vi "asynchronous safe state.vi"(9 "Module Info In":T1, 11 "Engine Tags In":T5) -> (1 "Module Info Out":T1, 3 "Engine Tags Out":T5)   [LabVIEW 2013, in "Standard Engine Runtime.lvclass"]
uses:
  Standard Engine Runtime.lvclass
  <vilib>/NI/Tag Bus/table/data table.ctl
  async execution info.ctl
  asynchronous process data.ctl
  async command notification.ctl
  <vilib>/NI/Tag Bus Module Framework/runtime/execution settings.ctl
  async error info.ctl
  <vilib>/NI/Tag Bus Module Framework/runtime/error classification.ctl
  Data Table with Transfer Spec.ctl
  <vilib>/NI/Tag Bus/table/transfer specification.ctl
  <vilib>/NI/Tag Bus/tag/Data Type.ctl
  Configuration/Module Decimation.ctl
  Configuration/Module Error Configuration.ctl
  Configuration/Error Actions By Category.ctl
  Configuration/Error Actions.ctl
  <vilib>/NI/Tag Bus/table/data table.lvlib
  <vilib>/NI/Tag Bus/tag/tag descriptor.lvclass
  Configuration/Standard Engine Configuration.lvclass
  <vilib>/NI/Tag Bus Module Framework/runtime/TBM module execution interface.lvclass
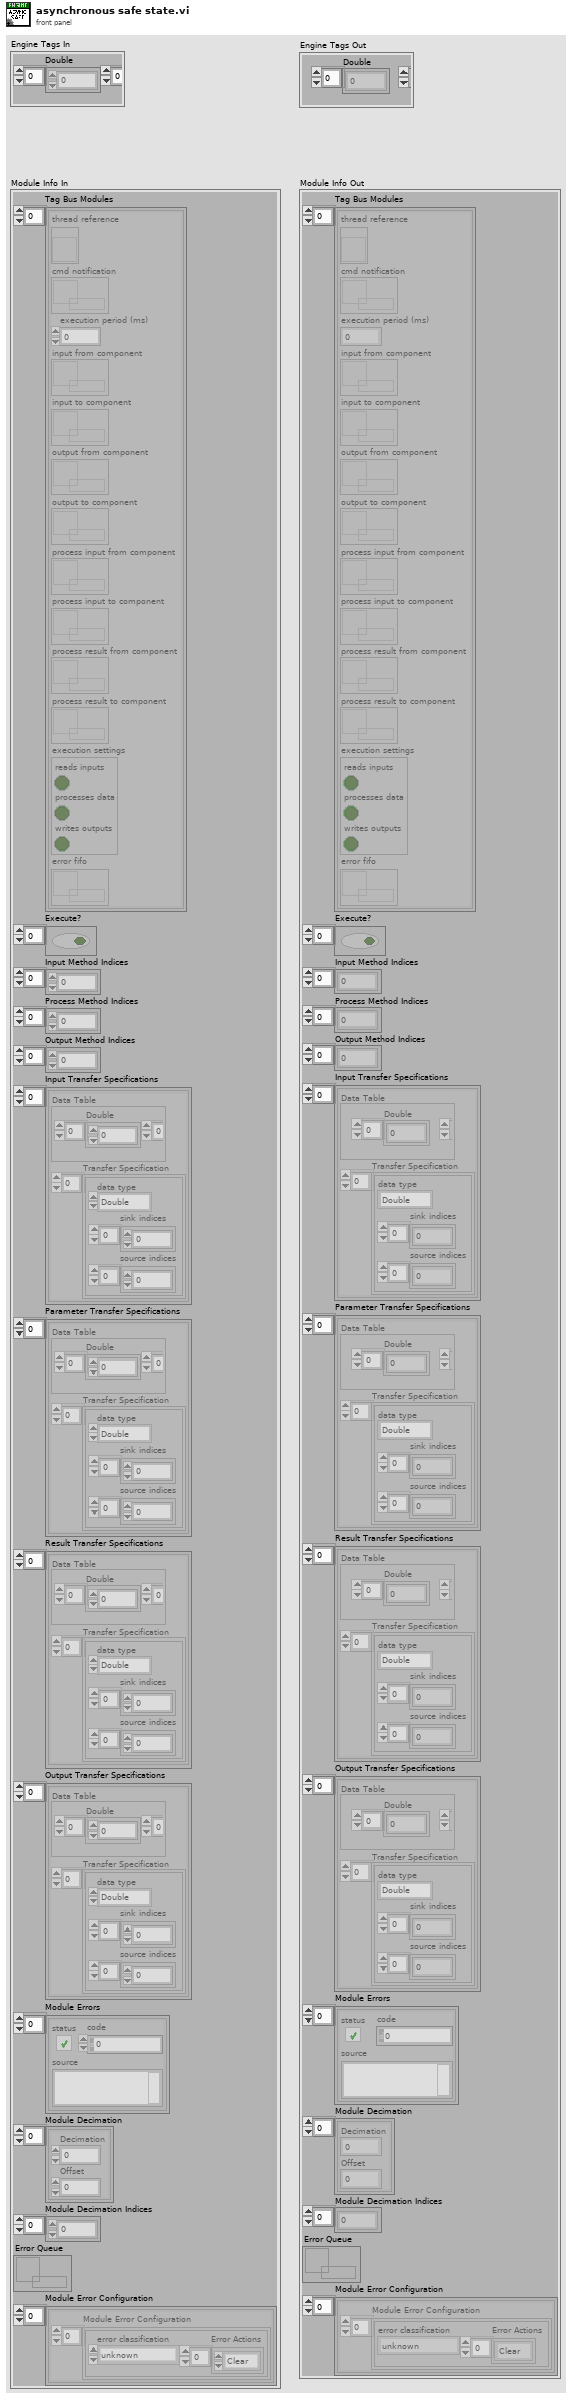
[diagram p1: front panel]
types:
  T1 = typedef "Standard Engine Runtime.lvclass/async execution info.ctl" = cluster{"Tag Bus Modules":T2[], "Execute?":bool[], "Input Method Indices":i32[], "Process Method Indices":i32[], "Output Method Indices":i32[], "Input Transfer Specifications":T4[], "Parameter Transfer Specifications":T4[], "Result Transfer Specifications":T4[], "Output Transfer Specifications":T4[], "Module Errors":errorcluster[], "Module Decimation":T8[], "Module Decimation Indices":i32[], "Error Queue":refnum<queue>, "Module Error Configuration":T9[]}
  T2 = typedef "Standard Engine Runtime.lvclass/asynchronous process data.ctl" = cluster{"thread reference":refnum<vi>, "cmd notification":refnum<k33>, "execution period (ms)":i32, "input from component":refnum<queue>, "input to component":refnum<queue>, "output from component":refnum<queue>, "output to component":refnum<queue>, "process input from component":refnum<queue>, "process input to component":refnum<queue>, "process result from component":refnum<queue>, "process result to component":refnum<queue>, "execution settings":T3, "error fifo":refnum<k33>}
  T3 = typedef "TBM module execution interface.lvclass/execution settings.ctl" = cluster{"reads inputs":bool, "processes data":bool, "writes outputs":bool}
  T4 = typedef "Standard Engine Runtime.lvclass/Data Table with Transfer Spec.ctl" = cluster{"Data Table":T5, "Transfer Specification":T6[]}
  T5 = typedef "tag bus.lvlib/data table.lvlib/data table.ctl" = cluster{"Double":dbl[], "Single":sgl[], "I64":i64[], "I32":i32[], "I16":i16[], "I8":i8[], "U64":u64[], "U32":u32[], "U16":u16[], "U8":u8[], "Boolean":bool[], "String":string[], "Array of Double":cluster{"DBL Array":dbl[]}[], "Array of Single":cluster{"SGL Array":sgl[]}[], "Array of I64":cluster{"I64 Array":i64[]}[], "Array of I32":cluster{"I32 Array":i32[]}[], "Array of I16":cluster{"I16 Array":i16[]}[], "Array of I8":cluster{"I8 Array":i8[]}[], "Array of U64":cluster{"U64 Array":u64[]}[], "Array of U32":cluster{"U32 Array":u32[]}[], "Array of U16":cluster{"U16 Array":u16[]}[], "Array of U8":cluster{"U8 Array":u8[]}[], "Array of Boolean":cluster{"Boolean Array":bool[]}[], "Array of String":cluster{"String Array":string[]}[]}
  T6 = typedef "tag bus.lvlib/data table.lvlib/transfer specification.ctl" = cluster{"data type":T7, "sink indices":i32[], "source indices":i32[]}
  T7 = typedef "tag bus.lvlib/tag descriptor.lvclass/Data Type.ctl" = enum16{"Double", "Single", "I64", "I32", "I16", "I8", "U64", "U32", "U16", "U8", "Boolean", "String", "Array of Double", "Array of Single", "Array of I64", "Array of I32", "Array of I16", "Array of I8", "Array of U64", "Array of U32", "Array of U16", "Array of U8", "Array of Boolean", "Array of String"}
  T8 = typedef "Standard Engine Configuration.lvclass/Module Decimation.ctl" = cluster{"Decimation":u16, "Offset":u16}
  T9 = typedef "Standard Engine Configuration.lvclass/Module Error Configuration.ctl" = cluster{"Module Error Configuration":T10[]}
  T10 = typedef "Standard Engine Configuration.lvclass/Error Actions By Category.ctl" = cluster{"error classification":T11, "Error Actions":T12[]}
  T11 = typedef "TBM module execution interface.lvclass/error classification.ctl" = enum16{"unknown", "none", "trivial", "recoverable", "critical"}
  T12 = typedef "Standard Engine Configuration.lvclass/Error Actions.ctl" = enum16{"Clear", "Notify", "Stop Component", "Stop Engine", "Safe State", "Attempt Recovery"}
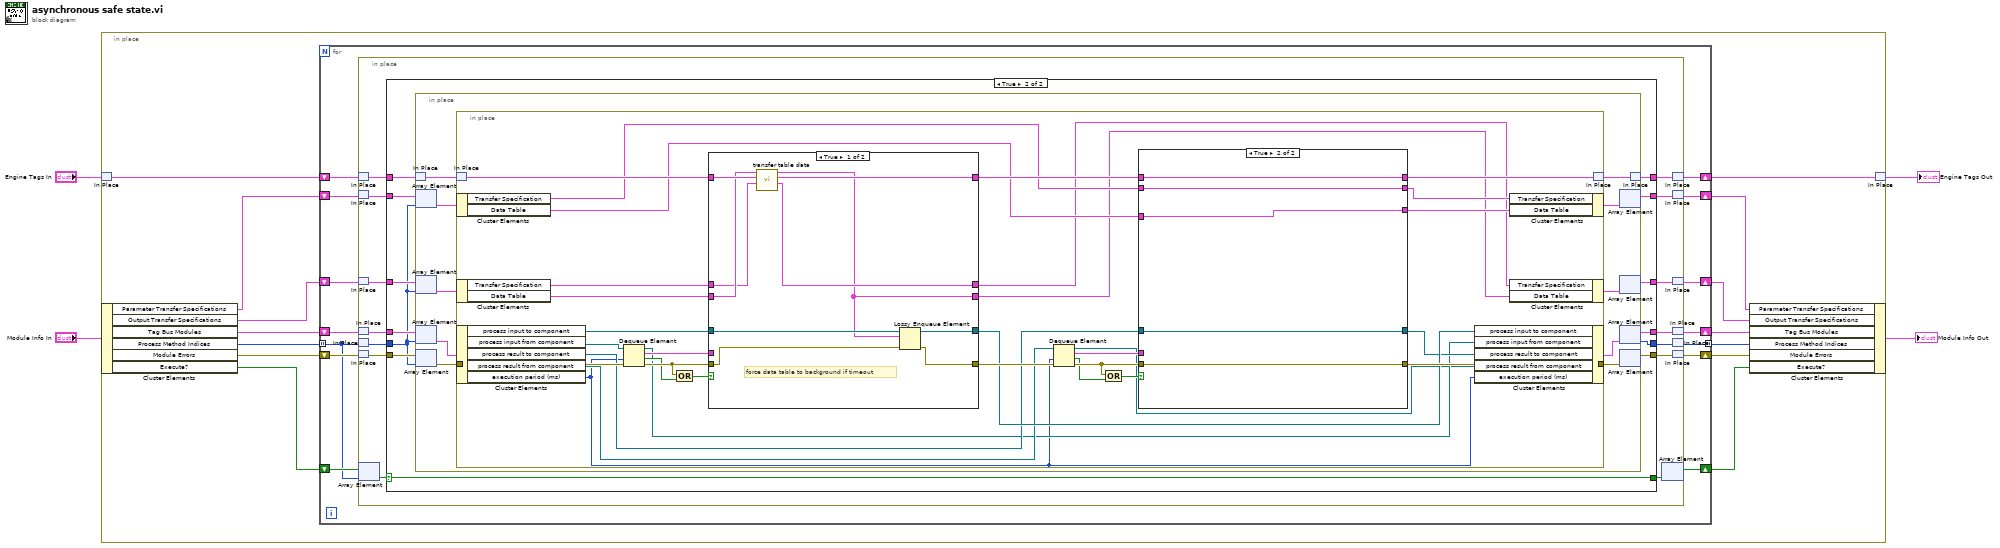
[diagram p0: block diagram]
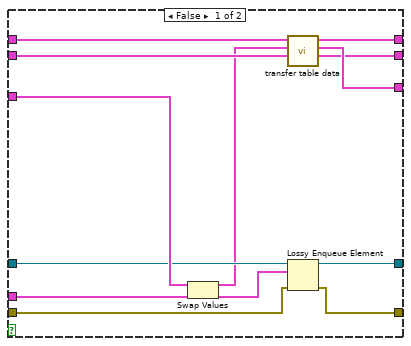
[diagram p3: hidden frame]
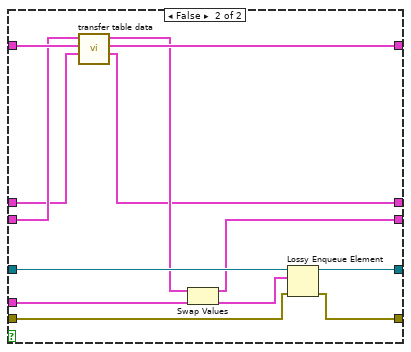
[diagram p4: hidden frame]
diagram:
  n1 = in-place {
    n2 = in-place-match #1("Engine Tags In") -> (w17:T5)
    n3 = in-place-cluster #2("Module Info In") -> ("Parameter Transfer Specifications"=w6:T4[], "Output Transfer Specifications"=w15:T4[], "Tag Bus Modules"=w12:T2[], "Process Method Indices"=w18:i32[], "Module Errors"=w14:errorcluster[], "Execute?"=w8:bool[])
    n4 = for {
      shift-right: [w25] -> w11
      shift-left: w12 -> [w26]
      tunnel: w18 -> [w22] mode=indexing
      shift-right: [w29] -> w16
      shift-left: w17 -> [w30]
      shift-right: [w27] -> w13
      shift-left: w15 -> [w28]
      shift-right: [w23] -> w10
      shift-left: w14 -> [w24]
      tunnel: [w21] -> w9 mode=indexing
      shift-right: [w31] -> w7
      shift-left: w8 -> [w32]
      shift-right: [w19] -> w5
      shift-left: w6 -> [w20]
      n5 = in-place {
        n6 = in-place-match #3(w30) -> (w44:T5)
        n7 = in-place-match #4(w20) -> (w33:T4[])
        n8 = in-place-match #5(w28) -> (w42:T4[])
        n9 = in-place-match #6(w26) -> (w40:T2[])
        n10 = in-place-match #7(w22) -> (w36:i32)
        n11 = in-place-match #8(w24) -> (w38:errorcluster[])
        n12 = in-place-array #9(w32, w22) -> (w46:bool)
        n13 = case shown="True" w46 {
          selector: w46 -> [w48 w57]
          tunnel: w44 -> [w53 w66]
          tunnel: [w53 w65] -> w43
          tunnel: w42 -> [w52 w64]
          tunnel: w40 -> [w51 w63]
          tunnel: w38 -> [w49 w62]
          tunnel: [w52 w61] -> w41
          tunnel: [w49 w60] -> w37
          tunnel: [w51 w59] -> w39
          tunnel: w36 -> [w50 w54]
          tunnel: [w50 w58] -> w35
          tunnel: [w48 w57] -> w45
          tunnel: [w47 w55] -> w34
          tunnel: w33 -> [w47 w56]
          frame False {
          }
          frame True {
            n14 = in-place {
              n15 = in-place-match #10(w66) -> (w76:T5)
              n16 = in-place-array #11(w56, w54) -> (w68:T4)
              n17 = in-place-array #12(w64, w54) -> (w74:T4)
              n18 = in-place-array #13(w63, w54) -> (w72:T2)
              n19 = in-place-array #14(w62, w54) -> (w70:errorcluster)
              n20 = in-place {
                in-place-border: w70 -> [w105]
                in-place-border: [w91] -> w69
                n21 = in-place-match #15(w76) -> (w107:T5)
                n22 = in-place-cluster #16(w68) -> ("Transfer Specification"=w96:T6[], "Data Table"=w93:T5)
                n23 = in-place-cluster #17(w74) -> ("Transfer Specification"=w106:T6[], "Data Table"=w104:T5)
                n24 = in-place-cluster #18(w72) -> ("process input to component"=w103:refnum<queue>, "process input from component"=w102:refnum<queue>, "process result to component"=w86:refnum<queue>, "process result from component"=w87:refnum<queue>, "execution period (ms)"=w82:i32)
                n25 = Dequeue Element(queue=w102, timeout in ms (-1)=w82, error in (no error)=w105) -> (queue out=w83:refnum<queue>, element=w84:T5, timed out?=w85:bool, error out=w100:errorcluster)
                n26 = Compound Arithmetic op=OR(w100, w85) -> (w101:bool)
                n27 = case shown="True" w101 {
                  tunnel: w107 -> [w131 w142]
                  tunnel: [w130 w141] -> w98
                  tunnel: [w126 w144] -> w90
                  tunnel: w106 -> [w128 w138]
                  tunnel: [w127 w137] -> w92
                  tunnel: w104 -> [w129 w140]
                  tunnel: w103 -> [w135 w148]
                  tunnel: [w134 w147] -> w89
                  tunnel: [w133 w146] -> w99
                  tunnel: w100 -> [w132 w145]
                  tunnel: w84 -> [_ w136]
                  frame True {
                    # "force data table to background if timeout"
                    n28 = call <vilib>:"transfer table data.vi"("transfer specification in"=w128, "data table source in"=w131, "data table sink in"=w129) -> ("transfer specification out"=w127:T6[], "data table source out"=w130:T5, "data table sink out"=w126:T5)  [unwired: 6 in]
                    n29 = Lossy Enqueue Element(queue=w135, element=w126, error in (no error)=w132) -> (queue out=w134:refnum<queue>, error out=w133:errorcluster)  [unwired: 2 out]
                  }
                  frame False {
                    n30 = call <vilib>:"transfer table data.vi"("transfer specification in"=w138, "data table source in"=w142, "data table sink in"=w140) -> ("transfer specification out"=w137:T6[], "data table source out"=w141:T5, "data table sink out"=w139:T5)  [unwired: 6 in]
                    n31 = Swap Values(12:w139, 14:w136) -> (1:w144:T5, 3:w143:T5)  [unwired: 1 in]
                    n32 = Lossy Enqueue Element(queue=w148, element=w143, error in (no error)=w145) -> (queue out=w147:refnum<queue>, error out=w146:errorcluster)  [unwired: 2 out]
                  }
                }
                n33 = Dequeue Element(queue=w87, timeout in ms (-1)=w82, error in (no error)=w99) -> (queue out=w77:refnum<queue>, element=w78:T5, timed out?=w79:bool, error out=w80:errorcluster)
                n34 = Compound Arithmetic op=OR(w80, w79) -> (w81:bool)
                n35 = case shown="True" w81 {
                  tunnel: w98 -> [w120 w121]
                  tunnel: [w119 w121] -> w97
                  tunnel: [w118 w123] -> w94
                  tunnel: w96 -> [w117 w122]
                  tunnel: [w116 w122] -> w95
                  tunnel: w93 -> [w115 w123]
                  tunnel: w86 -> [w114 w125]
                  tunnel: [w113 w125] -> w88
                  tunnel: [w112 w124] -> w91
                  tunnel: w80 -> [w108 w124]
                  tunnel: w78 -> [w110 _]
                  frame False {
                    n36 = Swap Values(12:w115, 14:w110) -> (1:w111:T5, 3:w109:T5)  [unwired: 1 in]
                    n37 = call <vilib>:"transfer table data.vi"("transfer specification in"=w117, "data table source in"=w111, "data table sink in"=w120) -> ("transfer specification out"=w116:T6[], "data table source out"=w118:T5, "data table sink out"=w119:T5)  [unwired: 6 in]
                    n38 = Lossy Enqueue Element(queue=w114, element=w109, error in (no error)=w108) -> (queue out=w113:refnum<queue>, error out=w112:errorcluster)  [unwired: 2 out]
                  }
                  frame True {
                  }
                }
                n39 = in-place-cluster #18("process input to component"=w89, "process input from component"=w83, "process result to component"=w88, "process result from component"=w77, "execution period (ms)"=w82) -> (w71:T2)
                n40 = in-place-cluster #16("Transfer Specification"=w95, "Data Table"=w94) -> (w67:T4)
                n41 = in-place-cluster #17("Transfer Specification"=w92, "Data Table"=w90) -> (w73:T4)
                n42 = in-place-match #15(w97) -> (w75:T5)
              }
              n43 = in-place-array #11(w67) -> (w55:T4[])  [unwired: 1 out]
              n44 = in-place-array #12(w73) -> (w61:T4[])  [unwired: 1 out]
              n45 = in-place-array #13(w71) -> (w59:T2[], w58:i32)
              n46 = in-place-array #14(w69) -> (w60:errorcluster[])  [unwired: 1 out]
              n47 = in-place-match #10(w75) -> (w65:T5)
            }
          }
        }
        n48 = in-place-array #9(w45) -> (w31:bool[])  [unwired: 1 out]
        n49 = in-place-match #3(w43) -> (w29:T5)
        n50 = in-place-match #4(w34) -> (w19:T4[])
        n51 = in-place-match #5(w41) -> (w27:T4[])
        n52 = in-place-match #6(w39) -> (w25:T2[])
        n53 = in-place-match #7(w35) -> (w21:i32)
        n54 = in-place-match #8(w37) -> (w23:errorcluster[])
      }
    }
    n55 = in-place-cluster #2("Parameter Transfer Specifications"=w5, "Output Transfer Specifications"=w13, "Tag Bus Modules"=w11, "Process Method Indices"=w9, "Module Errors"=w10, "Execute?"=w7) -> (→"Module Info Out":T1)
    n56 = in-place-match #1(w16) -> (→"Engine Tags Out":T5)
  }
